vi "Calculate If Swinging.vi"(2 "Swing Array Size":i32, 5 "IMU Ready":bool, 7 "Disable":bool, 10 "Swing Threshold":dbl, 11 "Yaw Pich Roll":cluster{"Yaw":dbl, "Pitch":dbl, "Roll":dbl}) -> (3 "Swinging Out":bool)   [LabVIEW 2023, in "PigeonIMU_SEN_ts.lvlib"]
uses:
  PigeonIMU_SEN_ts.lvlib
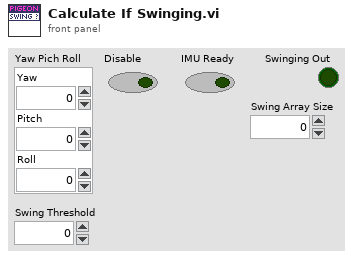
[diagram p1: front panel]
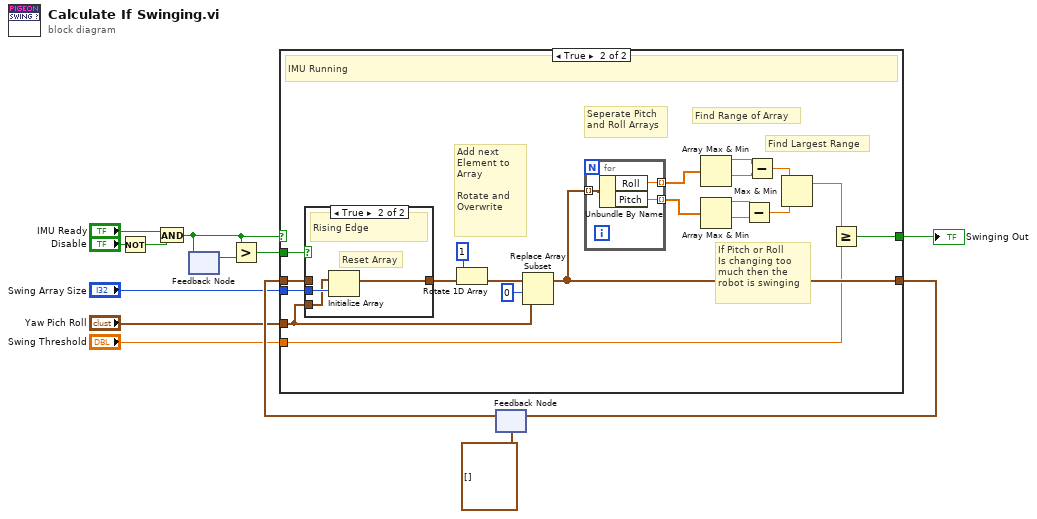
[diagram p0: block diagram]
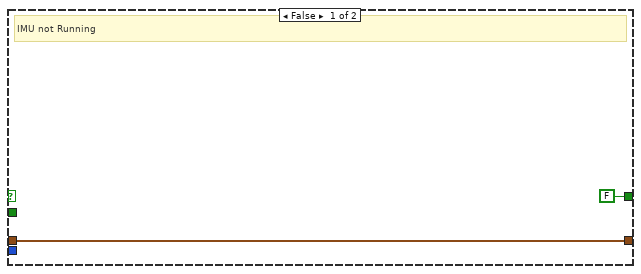
[diagram p2: hidden frame]
diagram:
  n1 = Not(x="Disable") -> (.not. x?=w1:bool)
  n2 = And(x="IMU Ready", y=w1) -> (x .and. y?=w7:bool)
  n3 = feedback-in #1(w7) -> ()
  n4 = feedback #1() -> (w8:bool)  [unwired: 1 in]
  n5 = Greater?(x=w7, y=w8) -> (0:w6:bool)
  n6 = feedback #2(cluster{"Yaw":dbl, "Pitch":dbl, "Roll":dbl}[] [] ("Yaw Pich Roll")) -> (w12:cluster{"Yaw":dbl, "Pitch":dbl, "Roll":dbl}[])
  n7 = case shown="True" w7 {
    tunnel: w12 -> [w15 w35]
    tunnel: "Swing Array Size" -> [_ w34]
    tunnel: w6 -> [_ w33]
    tunnel: "Yaw Pich Roll" -> [_ w29]
    tunnel: [w15 w27] -> w4
    tunnel: "Swing Threshold" -> [_ w17]
    tunnel: [FALSE w16] -> w2
    frame False {
      # "IMU not Running"
    }
    frame True {
      # "If Pitch or Roll\nIs changing too\nmuch then the \nrobot is swinging"
      # "Find Largest Range"
      # "Find Range of Array"
      # "Seperate Pitch\nand Roll Arrays"
      # "Add next\nElement to\nArray\n\nRotate and \nOverwrite"
      # "IMU Running"
      n8 = case shown="True" w33 {
        tunnel: w35 -> [w39 _]
        tunnel: w34 -> [_ w42]
        tunnel: [w39 w41] -> w31
        tunnel: w29 -> [_ w40]
        frame False {
          # "Keep Array"
          # "Not Rising Edge"
        }
        frame True {
          # "Reset Array"
          # "Rising Edge"
          n9 = Initialize Array(w40, w42) -> (w41:cluster{"Yaw":dbl, "Pitch":dbl, "Roll":dbl}[])
        }
      }
      n10 = Rotate 1D Array(1:w31, 2:1 ("n")) -> (0:w32:cluster{"Yaw":dbl, "Pitch":dbl, "Roll":dbl}[])
      n11 = Replace Array Subset(array=w32, new element=w29, index=0) -> (w27:cluster{"Yaw":dbl, "Pitch":dbl, "Roll":dbl}[])
      n12 = for {
        tunnel: w27 -> [w38] mode=indexing
        tunnel: [w37] -> w26 mode=indexing
        tunnel: [w36] -> w25 mode=indexing
        n13 = Unbundle By Name(w38) -> ("Roll"=w37:dbl, "Pitch"=w36:dbl)
      }
      n14 = Array Max & Min(array=w26) -> (max value=w24:dbl, min value=w23:dbl)  [unwired: 2 out]
      n15 = Array Max & Min(array=w25) -> (max value=w22:dbl, min value=w21:dbl)  [unwired: 2 out]
      n16 = Subtract(x=w22, y=w21) -> (x-y=w19:dbl)
      n17 = Subtract(x=w24, y=w23) -> (x-y=w20:dbl)
      n18 = Max & Min(x=w20, y=w19) -> (max(x,y)=w18:dbl)  [unwired: 1 out]
      n19 = Greater Or Equal?(x=w18, y=w17) -> (x >= y?=w16:bool)
    }
  }
  "Swinging Out" <- w2
  n20 = feedback-in #2(w4) -> ()
